vi "iterative_segments_to_centerline_oneiteration.vi"(7 "Segment Sequence Cluster Arrays":cluster{i32[]}[](array[cluster]), 8 "Potential Centerlines In":cluster{i32[]}[](array[cluster]), 9 "Potential Centerline Distances In":i32[](array[numeric]), 10 "Endpoints":i32[](array[numeric]), 11 "Concatenated Segments":i32[](array[numeric])) -> (0 "Potential Centerlines Out":cluster{i32[]}[](array[cluster]), 1 "Potential Centerline Lengths Out":i32[](array[numeric]), 2 "Timed Out":bool)   [LabVIEW 2019]
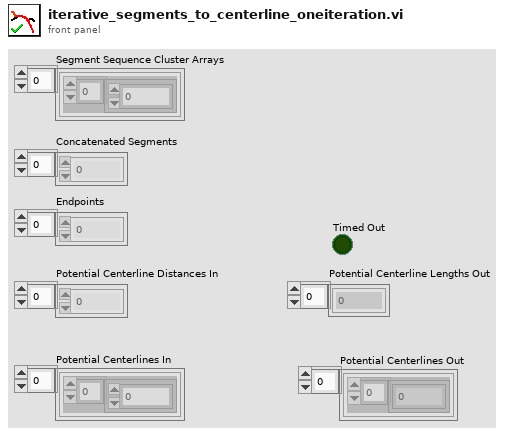
[diagram p1: front panel]
types:
  T1 = cluster{"Segment Sequence Cluster Arrays":cluster{i32[]}[]}
  T2 = cluster{"Segment Sequence Cluster Arrays":cluster{i32[]}[]}[]
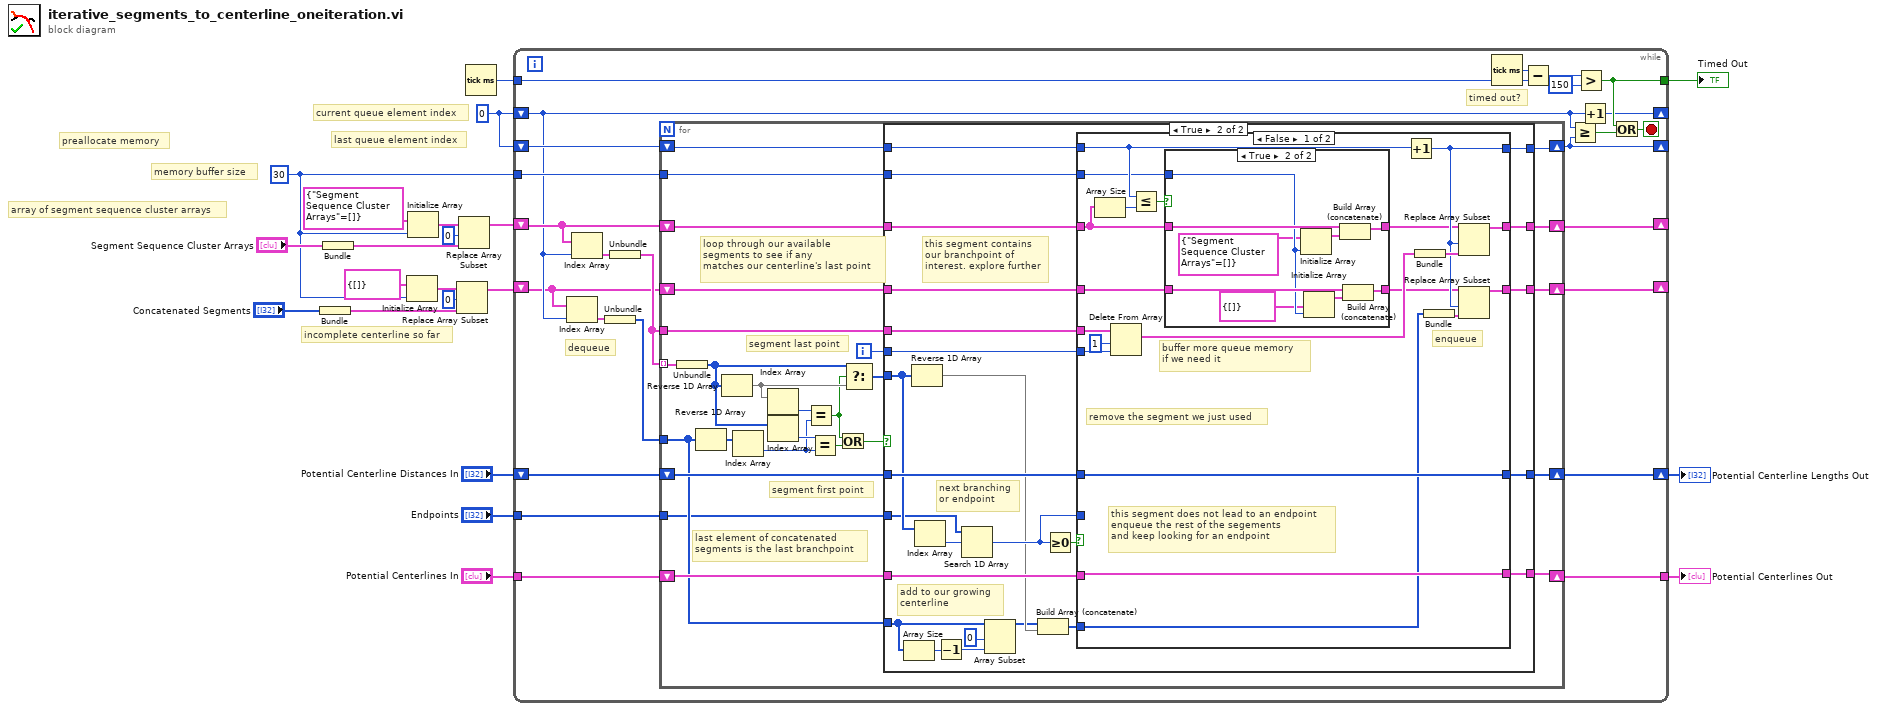
[diagram p0: block diagram]
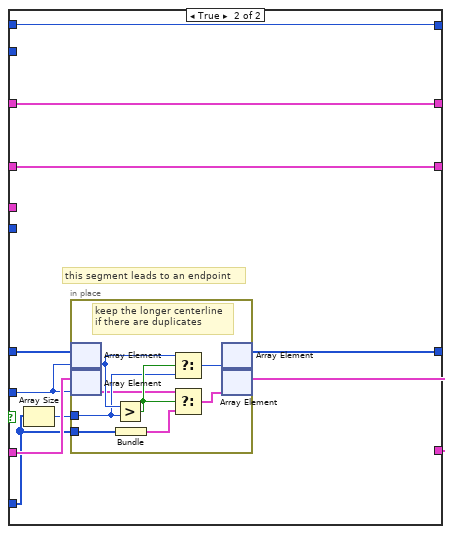
[diagram p4: hidden frame]
diagram:
  w6 = 30
  w12 = 0
  # "memory buffer size"
  # "preallocate memory"
  # "last queue element index"
  # "current queue element index"
  # "array of segment sequence cluster arrays"
  # "incomplete centerline so far"
  n1 = Bundle("Concatenated Segments"="Concatenated Segments") -> (w9:cluster{"Concatenated Segments":i32[]})  [unwired: 1 in]
  n2 = Bundle("Segment Sequence Cluster Arrays"="Segment Sequence Cluster Arrays") -> (w4:T1)  [unwired: 1 in]
  n3 = Initialize Array(cluster{"Concatenated Segments":i32[]} {"Concatenated Segments"=[]} ("output cluster"), w6) -> (w11:cluster{"Concatenated Segments":i32[]}[])
  n4 = Initialize Array(T1 {"Segment Sequence Cluster Arrays"=[]} ("output cluster"), w6) -> (w5:T2)
  n5 = Replace Array Subset(array=w11, new element=w9, index=0) -> (w8:cluster{"Concatenated Segments":i32[]}[])
  n6 = Replace Array Subset(array=w5, new element=w4, index=0) -> (w7:T2)
  n7 = Tick Count (ms)() -> (millisecond timer value=w19:u32)
  n8 = while {
    shift-right: [w45] -> w20
    shift-left: "Potential Centerline Distances In" -> [w46]
    shift-right: [w44] -> _
    shift-left: w7 -> [w29]
    tunnel: w19 -> [w40]
    tunnel: [w38] -> w18
    tunnel: "Potential Centerlines In" -> [w37]
    tunnel: [w36] -> w16
    shift-right: [w31] -> _
    shift-left: w8 -> [w22]
    tunnel: "Endpoints" -> [w30]
    shift-right: [w27] -> _
    shift-left: w12 -> [w23]
    shift-right: [w25] -> _
    shift-left: w12 -> [w28]
    tunnel: w6 -> [w24]
    stop <- w39 stop-if-true
    # "timed out?"
    # "dequeue"
    n9 = Index Array(array=w22, index=w23) -> (element=w34:cluster{"Concatenated Segments":i32[]})
    n10 = Index Array(array=w29, index=w23) -> (element=w33:T1)
    n11 = Unbundle(w34) -> ("Concatenated Segments"=w35:i32[])
    n12 = Unbundle(w33) -> ("Segment Sequence Cluster Arrays"=w32:cluster{i32[]}[])
    n13 = for {
      tunnel: w32 -> [w72] mode=indexing
      tunnel: w35 -> [w57]
      tunnel: w32 -> [w63]
      shift-right: [w55] -> w45
      shift-left: w46 -> [w61]
      shift-right: [w56] -> w36
      shift-left: w37 -> [w60]
      shift-right: [w53] -> w44
      shift-left: w29 -> [w54]
      shift-right: [w51] -> w31
      shift-left: w22 -> [w52]
      tunnel: w30 -> [w50]
      shift-right: [w48] -> w25
      shift-left: w28 -> [w49]
      tunnel: w24 -> [w47]
      i -> [w62]
      # "loop through our available \nsegments to see if any\nmatches our centerline's last point"
      # "last element of concatenated\nsegments is the last branchpoint"
      # "segment first point"
      # "segment last point"
      n14 = Unbundle(w72) -> (w68:i32[])
      n15 = Reverse 1D Array(array=w57) -> (reversed array=w59:i32[])
      n16 = Reverse 1D Array(array=w68) -> (reversed array=w69:i32[])
      n17 = Index Array(array=w59) -> (element=w58:i32)  [unwired: 1 in]
      n18 = Index Array(array=w69) -> (element=w70:i32)  [unwired: 1 in]
      n19 = Index Array(array=w68) -> (element=w71:i32)  [unwired: 1 in]
      n20 = Equal?(x=w70, y=w58) -> (x = y?=w65:bool)
      n21 = Equal?(x=w71, y=w58) -> (x = y?=w67:bool)
      n22 = Or(x=w65, y=w67) -> (x .or. y?=w66:bool)
      n23 = Select(t=w68, s=w65, f=w69) -> (s? t:f=w64:i32[])
      n24 = case shown="True" w66 {
        tunnel: w64 -> [_ w90]
        tunnel: w63 -> [_ w95]
        tunnel: w62 -> [_ w94]
        tunnel: w61 -> [w77 w100]
        tunnel: w60 -> [w76 w98]
        tunnel: w57 -> [_ w88]
        tunnel: [w76 w97] -> w56
        tunnel: [w77 w96] -> w55
        tunnel: w54 -> [w75 w85]
        tunnel: [w75 w84] -> w53
        tunnel: w52 -> [w74 w83]
        tunnel: [w74 w82] -> w51
        tunnel: w50 -> [_ w81]
        tunnel: w49 -> [w73 w80]
        tunnel: [w73 w79] -> w48
        tunnel: w47 -> [_ w78]
        frame False {
          # "this segment does not contain our branchpoint of interest. leave it be."
        }
        frame True {
          # "add to our growing\ncenterline"
          # "this segment contains\nour branchpoint of\ninterest. explore further"
          # "next branching\nor endpoint"
          n25 = Array Size(array=w88) -> (size(s)=w86:i32)
          n26 = Reverse 1D Array(array=w90) -> (reversed array=w93:i32[])
          n27 = Index Array(array=w90) -> (element=w102:i32)  [unwired: 1 in]
          n28 = Decrement(x=w86) -> (x-1=w87:i32)
          n29 = Search 1D Array(1D array=w81, element=w102) -> (index of element=w99:i32)  [unwired: 1 in]
          n30 = Array Subset(array=w88, index=0 ("length"), length=w87) -> (w89:i32[])
          n31 = Build Array (concatenate)(w89, w93) -> (w92:i32[])
          n32 = Greater Or Equal To 0?(x=w99) -> (x >= 0?=w101:bool)
          n33 = case shown="False" w101 {
            tunnel: w100 -> [w118 w143]
            tunnel: w99 -> [_ w141]
            tunnel: w98 -> [w119 w142]
            tunnel: [w119 w139] -> w97
            tunnel: [w118 w138] -> w96
            tunnel: w95 -> [w122 _]
            tunnel: w94 -> [w120 _]
            tunnel: w92 -> [w114 w137]
            tunnel: w85 -> [w107 w136]
            tunnel: [w117 w136] -> w84
            tunnel: w83 -> [w105 w135]
            tunnel: [w115 w135] -> w82
            tunnel: w80 -> [w109 w134]
            tunnel: [w111 w134] -> w79
            tunnel: w78 -> [w103 _]
            frame False {
              # "buffer more queue memory\nif we need it"
              # "enqueue"
              # "remove the segment we just used"
              # "this segment does not lead to an endpoint\nenqueue the rest of the segements \nand keep looking for an endpoint"
              n34 = Array Size(array=w107) -> (size(s)=w110:i32)
              n35 = Delete From Array(array=w122, length=1, index=w120) -> (array with subset deleted=w116:cluster{i32[]}[])  [unwired: 1 out]
              n36 = Less Or Equal?(x=w109, y=w110) -> (x <= y?=w108:bool)
              n37 = case shown="True" w108 {
                tunnel: w107 -> [w124 w133]
                tunnel: [w124 w132] -> w106
                tunnel: w105 -> [w123 w131]
                tunnel: [w123 w130] -> w104
                tunnel: w103 -> [_ w127]
                frame False {
                }
                frame True {
                  n38 = Initialize Array(T1 {"Segment Sequence Cluster Arrays"=[]} ("output cluster"), w127) -> (w129:T2)
                  n39 = Initialize Array(cluster{"Concatenated Segments":i32[]} {"Concatenated Segments"=[]} ("output cluster"), w127) -> (w128:cluster{"Concatenated Segments":i32[]}[])
                  n40 = Build Array (concatenate)(w133, w129) -> (w132:T2)
                  n41 = Build Array (concatenate)(w131, w128) -> (w130:cluster{"Concatenated Segments":i32[]}[])
                }
              }
              n42 = Increment(x=w109) -> (x+1=w111:i32)
              n43 = Bundle("Segment Sequence Cluster Arrays"=w116) -> (w113:T1)  [unwired: 1 in]
              n44 = Bundle(w114) -> (w112:cluster{i32[]})  [unwired: 1 in]
              n45 = Replace Array Subset(array=w106, new element=w113, index=w111) -> (w117:T2)
              n46 = Replace Array Subset(array=w104, new element=w112, index=w111) -> (w115:cluster{"Concatenated Segments":i32[]}[])
            }
            frame True {
              # "this segment leads to an endpoint"
              n47 = Array Size(array=w137) -> (size(s)=w140:i32)
              n48 = in-place {
                in-place-border: w140 -> [w147]
                in-place-border: w137 -> [w144]
                # "keep the longer centerline\nif there are duplicates"
                n49 = in-place-array #1(w143, w141) -> (w151:i32)
                n50 = in-place-array #2(w142, w141) -> (w146:cluster{i32[]})
                n51 = Greater?(x=w151, y=w147) -> (0:w150:bool)
                n52 = Bundle(w144) -> (w145:cluster{i32[]})  [unwired: 1 in]
                n53 = Select(t=w151, s=w150, f=w147) -> (s? t:f=w148:i32)
                n54 = Select(t=w146, s=w150, f=w145) -> (s? t:f=w149:cluster{i32[]})
                n55 = in-place-array #1(w148) -> (w138:i32[])  [unwired: 1 out]
                n56 = in-place-array #2(w149) -> (w139:cluster{i32[]}[])  [unwired: 1 out]
              }
            }
          }
        }
      }
    }
    n57 = Tick Count (ms)() -> (millisecond timer value=w43:u32)
    n58 = Subtract(x=w43, y=w40) -> (x-y=w42:u32)
    n59 = Greater Or Equal?(x=w23, y=w25) -> (x >= y?=w26:bool)
    n60 = Greater?(x=w42, y=u32 150) -> (0:w38:bool)
    n61 = Increment(x=w23) -> (x+1=w27:i32)
    n62 = Or(x=w38, y=w26) -> (x .or. y?=w39:bool)
  }
  "Potential Centerline Lengths Out" <- w20
  "Timed Out" <- w18
  "Potential Centerlines Out" <- w16
